vi "Convert TickNum to XY (FPGA).vi"(0 "numAcqTick":fxp<+,32,32>) -> (1 "PixelXArray":fxp<+,1,1>[](array[numeric]), 2 "PixelY":fxp<+,12,12>=1.0)   [LabVIEW 2013, in "FPGA Image Processing.lvlib"]
uses:
  FPGA Image Processing.lvlib
  <vilib>/rvi/FXPMathLib/FxpDiv/subVIs/nifxpmath_Div_SimConfig.ctl
  <vilib>/rvi/FXPMathLib/FxpDiv/simVIs/DllFxpDivTemp_sub.vi
  <vilib>/rvi/FXPMathLib/FxpDiv/XNode/nifxpmath_Div.xnode
  <vilib>/rvi/FXPMathLib/FxpMul/XNode/nifxpmath_Multiplier.xnode
  <vilib>/rvi/FXPMathLib/FxpSub/XNode/nifxpmath_Sub.xnode
  <vilib>/rvi/FXPMathLib/sim/FxpSim.dll
panel:
  out "output valid":bool
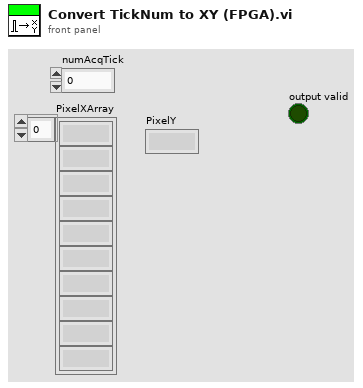
[diagram p1: front panel]
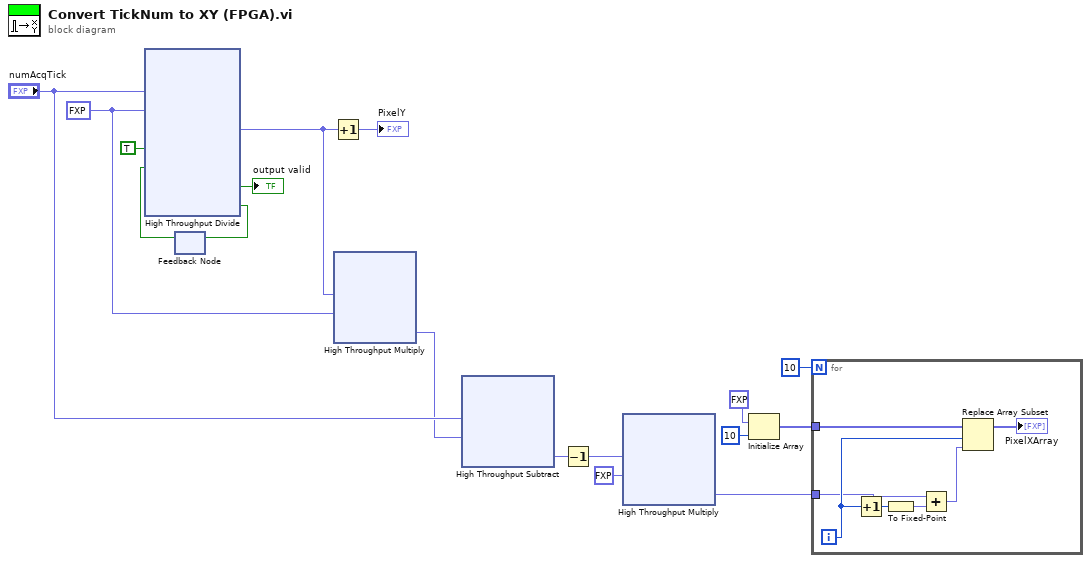
[diagram p0: block diagram]
diagram:
  w14 = fxp<+,8,8> 204.0 ("y")
  n1 = feedback #1() -> (w1:bool)  [unwired: 1 in]
  n2 = xnode "High Throughput Divide"("x"="numAcqTick", "y"=w14, "input valid"=TRUE, "ready for output (T)"=w1) -> ("x/y"=w15:fxp<+,11,11>, "output valid"=→"output valid":bool, "ready for input"=w2:bool)
  n3 = feedback-in #1(w2) -> ()
  n4 = Increment(x=w15) -> (x+1=→"PixelY":fxp<+,12,12>)
  n5 = xnode "High Throughput Multiply"("x"=w15, "y"=w14) -> ("x*y"=w13:fxp<+,19,19>)
  n6 = xnode "High Throughput Subtract"("x"="numAcqTick", "y"=w13) -> ("x-y"=w12:fxp<+/-,34,34>)
  n7 = Decrement(x=w12) -> (x-1=w10:fxp<+/-,35,35>)
  n8 = xnode "High Throughput Multiply"("x"=w10, "y"=fxp<+,4,4> 10.0) -> ("x*y"=w6:fxp<+/-,39,39>)
  n9 = Initialize Array(fxp<+,1,1> 0.0 ("element"), 10 ("dimension size")) -> (w7:fxp<+,1,1>[])
  n10 = for {
    N: 10 -> [_]
    tunnel: w7 -> [w24]
    tunnel: w6 -> [w22]
    i -> [w23]
    n11 = Increment(x=w23) -> (x+1=w21:i32)
    n12 = To Fixed-Point(number=w21) -> (fixed-point=w20:fxp<+/-,32,32>)  [unwired: 1 in]
    n13 = Add(x=w22, y=w20) -> (x+y=w19:fxp<+/-,40,40>)
    n14 = Replace Array Subset(array=w24, new element=w19, index=w23) -> (→"PixelXArray":fxp<+,1,1>[])
  }
